vi "SetVCLKReg.vi"(1 "vfreq":u8, 2 "lines":u32) -> ()   [LabVIEW 2014]
uses:
  ESLSCDLL.dll
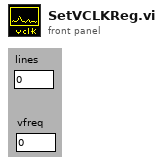
[diagram p1: front panel]
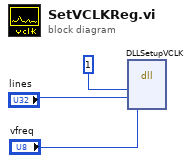
[diagram p0: block diagram]
diagram:
  n1 = dll-call lib="C:/Users/Gerhard/Documents/New64/lv/1cam/board.vis/ESLSCDLL.dll" fn="DLLSetupVCLK"("drv"=u32 1, "lines"="lines", "vfreq"="vfreq") -> ()  [unwired: 7 in, 2 out]
